vi "Section File Open.vi"(8 "error in (no error)":errorcluster, 11 "Section File Path":path) -> (0 "error out":errorcluster, 3 "Section Reference out":u64 format="%.0x")   [LabVIEW 2013, in "Hierarchy Framework.lvlib" / "Section.lvclass"]
doc: "Open user define section file,it return a <b>Section Reference</b>."
uses:
  Section.lvclass
  Generic/Generic.lvclass
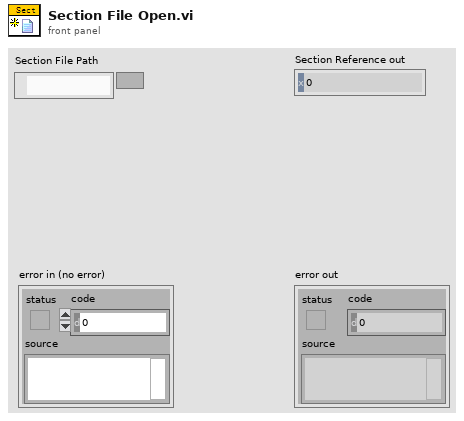
[diagram p1: front panel]
types:
  T1 = enum16{"open", "replace", "create", "open or create", "replace or create", "replace or create with confirmation"}
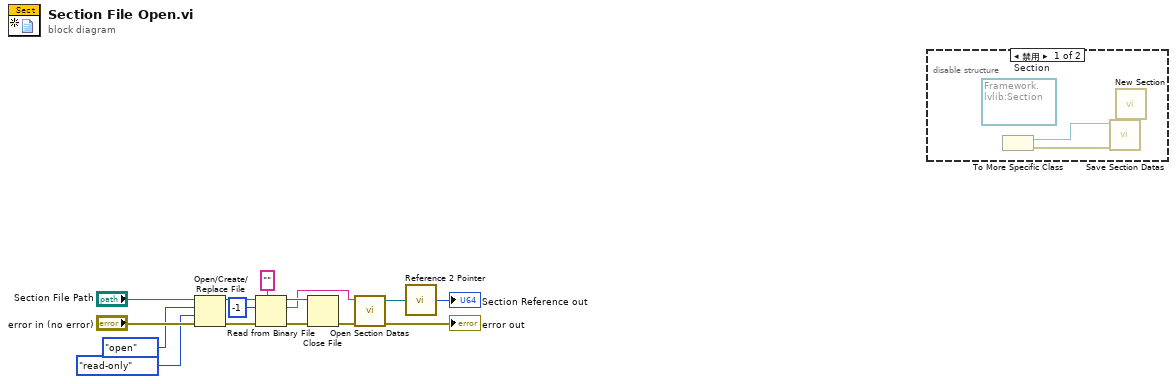
[diagram p0: block diagram]
diagram:
  n1 = Open/Create/Replace File(file path (use dialog)="Section File Path", error in="error in (no error)", operation (0:open)=T1."open" ("操作(0:open)"), access (0:read/write)=enum16{"read/write", "read-only", "write-only"}."read-only" ("权限(0:read/write)")) -> (refnum out=w10:refnum<file>, error out=w11:errorcluster)  [unwired: 2 in, 1 out]
  n2 = Read from Binary File(7:"", 8:w11, 10:-1 ("总数(1)"), 11:w10) -> (0:w9:errorcluster, 2:w2:string, 3:w8:refnum<file>)  [unwired: 2 in, 1 out]
  n3 = Close File(refnum=w8, error in=w9) -> (error out=w3:errorcluster)  [unwired: 1 out]
  n4 = call "Open Section Datas.vi"("error in (no error)"=w3, "Data in"=w2) -> ("error out"=→"error out":errorcluster, "Section"=w5:refnum<data-value>)  [unwired: 8 in]
  n5 = call "Reference 2 Pointer.vi"("Generic Reference"=w5) -> ("Pointer"=→"Section Reference out":u64)  [unwired: 1 out]
  n6 = disable-structure shown="禁用" {
    frame Disabled {
      (unwired) refnum<data-value> refnum  # Section
      n7 = To More Specific Class() -> (specific class reference=w17:refnum<data-value>, error out=w16:errorcluster)  [unwired: 3 in]
      n8 = call "Save Section Datas.vi"("error in (no error)"=w16, "Section in"=w17) -> ()  [unwired: 7 in, 3 out]
      n9 = call "New Section.vi"() -> ()  [unwired: 10 in, 2 out]
    }
    frame Enabled {
    }
  }
